vi "Package整体图.vi"() -> ()   [LabVIEW 2014]
panel:
  in  "Add":bool
  in  "Zip":bool
  in  "Package":bool
  in  "Java":bool
  in  "Box":bool
  in  "Black":bool
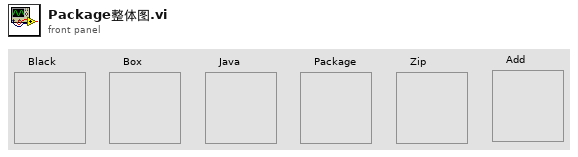
[diagram p1: front panel]
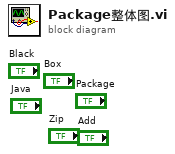
[diagram p0: block diagram]
diagram:
